vi "Pre Launch Init.vi"(11 "Controller in":refnum<class "Controller.lvclass">) -> (0 "error out":errorcluster, 3 "Controller out":refnum<class "Controller.lvclass">)   [LabVIEW 2026, in "Controller Actor.lvlib" / "Controller.lvclass"]
doc: "(<B>Filename</B>: Actor Framework.lvlib:Actor.lvclass:Pre Launch Init.vi)\n\nDefines behavior that occurs after the Launch Actor method is invoked but before the actor's Actor Core method begins running.\n\nThe Pre Launch Init method is guaranteed to finish before the Launch Actor method returns to its caller and before the actor itself receives any messages. Any references that the Pre Launch Init method obtains are guaranteed to have the same lifetime as the actor itself. Any errors that the Pre Launch Init method returns will abort the launch.\n\nBy default, this method does nothing. A descendant class may override it to define behavior."
uses:
  Controller.lvclass
  Controller.lvclass/Controller.ctl
  <vilib>/ActorFramework/Actor/Actor.lvclass
  configuration/Configuration.lvclass
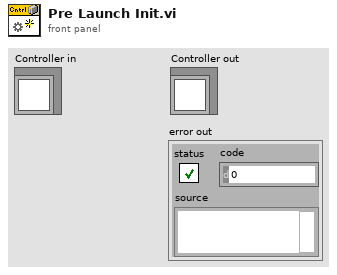
[diagram p1: front panel]
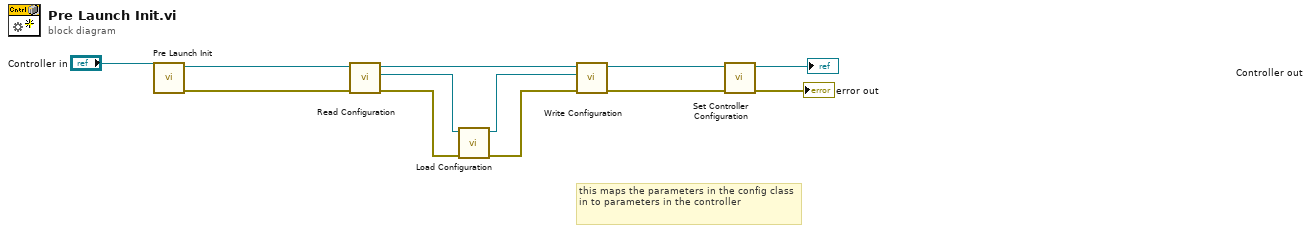
[diagram p0: block diagram]
diagram:
  # "this maps the parameters in the config class in to parameters in the controller"
  n1 = call-parent "Pre Launch Init.vi"("Actor in"="Controller in") -> ("error out"=w3:errorcluster, "Actor out"=w4:refnum<class "Controller.lvclass">)  [unwired: 9 in]
  n2 = call "Read Configuration.vi"("error in (no error)"=w3, "Controller in"=w4) -> ("error out"=w10:errorcluster, "Configuration.lvlib:Configuration.lvclass"=w11:refnum<class "Configuration.lvclass">, "Controller out"=w7:refnum<class "Controller.lvclass">)  [unwired: 7 in]
  n3 = call "Load Configuration.vi"("error in (no error)"=w10, "Configuration in"=w11) -> ("error out"=w8:errorcluster, "Configuration out"=w9:refnum<class "Configuration.lvclass">)  [unwired: 7 in, 1 out]
  n4 = call "Write Configuration.vi"("error in (no error)"=w8, "Configuration.lvlib:Configuration.lvclass"=w9, "Controller in"=w7) -> ("error out"=w1:errorcluster, "Controller out"=w2:refnum<class "Controller.lvclass">)  [unwired: 7 in]
  n5 = call-dynamic "Set Controller Configuration.vi"("error in (no error)"=w1, "Controller in"=w2) -> ("error out"=→"error out":errorcluster, "Controller out"=→"Controller out":refnum<class "Controller.lvclass">)  [unwired: 8 in]
